vi "EMG_Threshold_Calibration.vi"(0 "Biceps harder contraction threshold in (V)":dbl, 1 "Biceps contraction threshold in (V)":dbl, 2 "System calibrated? (input)":bool, 3 "Calibrate?":bool, 5 "Biceps EMG signal (V)":dbl[](array[numeric]), 9 "Triceps EMG signal (V)":dbl[](array[numeric]), 12 "Triceps contraction threshold in (V)":dbl, 14 "Triceps harderd contraction threshold in (V)":dbl) -> (4 "Biceps contraction threshold out (V)":dbl, 6 "Triceps contraction threshold out (V)":dbl, 8 "System calibrated?":bool, 10 "Triceps harderd contraction threshold out (V)":dbl, 15 "Biceps harder contraction threshold out (V)":dbl)   [LabVIEW 2015]
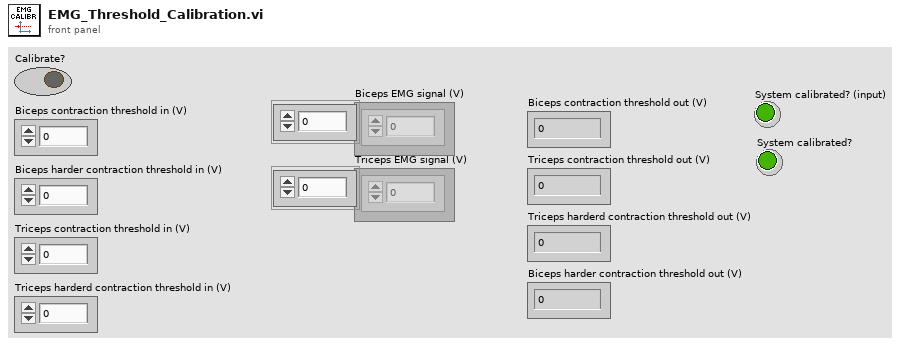
[diagram p1: front panel]
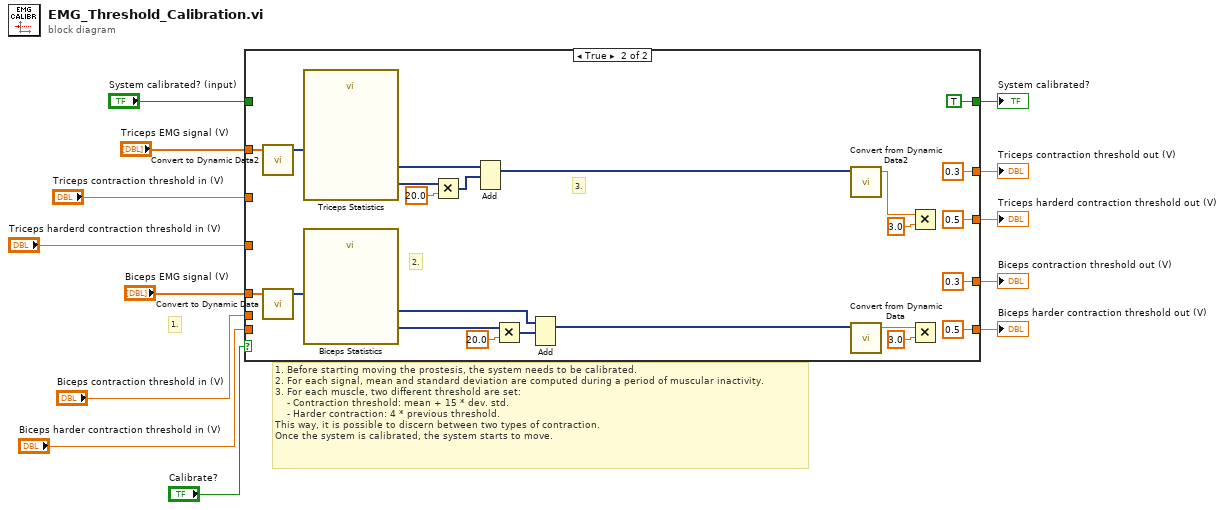
[diagram p0: block diagram]
diagram:
  # "1."
  # "1. Before starting moving the prostesis, the system needs to be calibrated.\n2. For each signal, mean and standard deviation are computed during a period of muscular inactivity.\n3. For each muscle, two different threshold are set:\n    - Contraction threshold: mean + 15 * dev. std.\n    - Harder contraction: 4 * previous threshold.\nThis way, it is possible to discern between two types of contraction.\nOnce the system is calibrated, the system starts to move."
  n1 = case shown="True" "Calibrate?" {
    tunnel: "Biceps EMG signal (V)" -> [_ w41]
    tunnel: [w18 0.3 ("Biceps contraction threshold in (V)")] -> w4
    tunnel: "Biceps contraction threshold in (V)" -> [w18 _]
    tunnel: [w17 0.5 ("Biceps harder contraction threshold in (V)")] -> w13
    tunnel: "Biceps harder contraction threshold in (V)" -> [w17 _]
    tunnel: "Triceps EMG signal (V)" -> [_ w28]
    tunnel: [w16 0.3 ("Triceps contraction threshold in (V)")] -> w11
    tunnel: "Triceps contraction threshold in (V)" -> [w16 _]
    tunnel: [w15 0.5 ("Triceps harderd contraction threshold in (V)")] -> w12
    tunnel: "Triceps harderd contraction threshold in (V)" -> [w15 _]
    tunnel: [w14 TRUE] -> w2
    tunnel: "System calibrated? (input)" -> [w14 _]
    frame False {
    }
    frame True {
      # "3."
      # "2."
      n2 = call "Convert to Dynamic Data2"("Array"=w28) -> ("Dynamic Data Type"=w34:dynamicdata)  [unwired: 3 in]
      n3 = call "Convert to Dynamic Data"("Array"=w41) -> ("Dynamic Data Type"=w40:dynamicdata)  [unwired: 3 in]
      n4 = call "Triceps Statistics"("Signals"=w34) -> ("Standard Dev"=w30:dynamicdata, "Arithmetic Mean"=w29:dynamicdata)  [unwired: 24 in, 1 out]
      n5 = call "Biceps Statistics"("Signals"=w40) -> ("Standard Dev"=w36:dynamicdata, "Arithmetic Mean"=w35:dynamicdata)  [unwired: 24 in, 1 out]
      n6 = Multiply(x=w30, y=20.0) -> (x*y=w32:dynamicdata)
      n7 = Add(1:w32, 2:w29) -> (0:w31:dynamicdata)  [unwired: 1 in, 1 out]
      n8 = Multiply(x=w36, y=20.0) -> (x*y=w38:dynamicdata)
      n9 = Add(1:w38, 2:w35) -> (0:w37:dynamicdata)  [unwired: 1 in, 1 out]
      n10 = call "Convert from Dynamic Data2"("Dynamic Data Type"=w31) -> ("Scalar"=w24:dbl)  [unwired: 3 in]
      n11 = call "Convert from Dynamic Data"("Dynamic Data Type"=w37) -> ("Scalar"=w27:dbl)  [unwired: 3 in]
      n12 = Multiply(x=w24, y=3.0) -> ()  [unwired: 1 out]
      n13 = Multiply(x=w27, y=3.0) -> ()  [unwired: 1 out]
    }
  }
  "Biceps harder contraction threshold out (V)" <- w13
  "Triceps harderd contraction threshold out (V)" <- w12
  "Triceps contraction threshold out (V)" <- w11
  "Biceps contraction threshold out (V)" <- w4
  "System calibrated?" <- w2
